vi "_builtins_arrange_object.vi"(8 "error in (no error)":errorcluster, 10 "Arrange":T1, 11 "GObject in":refnum<vi>) -> (0 "error out":errorcluster, 2 "object arranged?":bool, 3 "GObject out":refnum<vi>)   [LabVIEW 2019, in "Script.lvlib"]
doc: "Arranges the selected block diagram objects vertically to align the source terminal to the adjacent sink terminal (left-to-right) or sink to source terminals (right-to-left).\n\nCreated by: Ryan Pacini"
uses:
  Script.lvlib
  _builtins_arrange.ctl
  _builtins_label_position.ctl
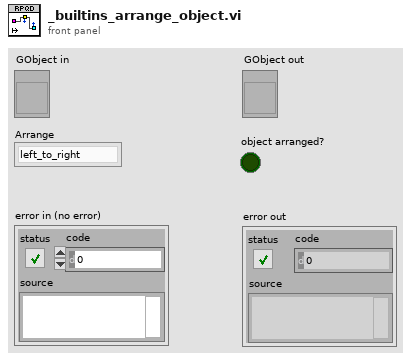
[diagram p1: front panel]
types:
  T1 = typedef "Script.lvlib/_builtins_arrange.ctl" = enum8{"left_to_right", "right_to_left"}
  T2 = typedef "Script.lvlib/_builtins_label_position.ctl" = enum8{"Unchanged", "Top-left", "Top-middle", "Top-right", "Right-top", "Right-middle", "Right-bottom", "Bottom-right", "Bottom-middle", "Bottom-left", "Left-bottom", "Left-middle", "Left-top"}
  T3 = typedef "LVRectTypeDef.ctl" = cluster{"Left":i16, "Top":i16, "Right":i16, "Bottom":i16}
  T4 = cluster{"Position":cluster{"h":i16, "v":i16}, "Flags":i32, "Type":enum32{"LooseEnd", "Endpoint", "Bend", "Junction"}, "Up Joint Index":i16, "Down Joint Index":i16, "Left Joint Index":i16, "Right Joint Index":i16}[]
  T5 = typedef "LVPositionTypeDef.ctl" = cluster{"Left":i32, "Top":i32}
  T6 = cluster{"Left":i32, "Top":i32, "Right":i32, "Bottom":i32}
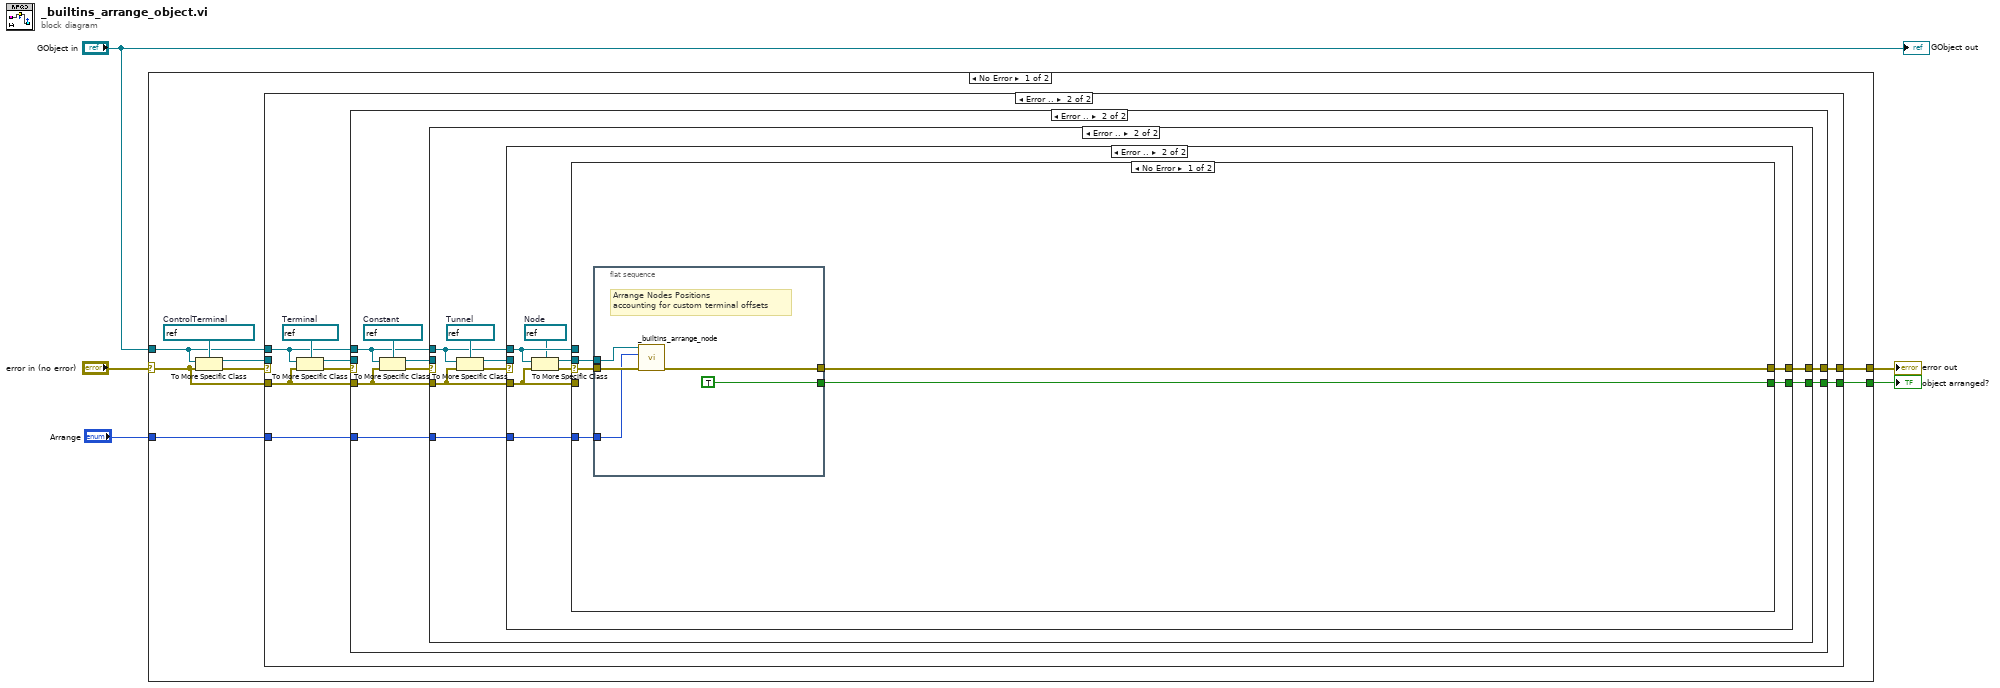
[diagram p0: block diagram]
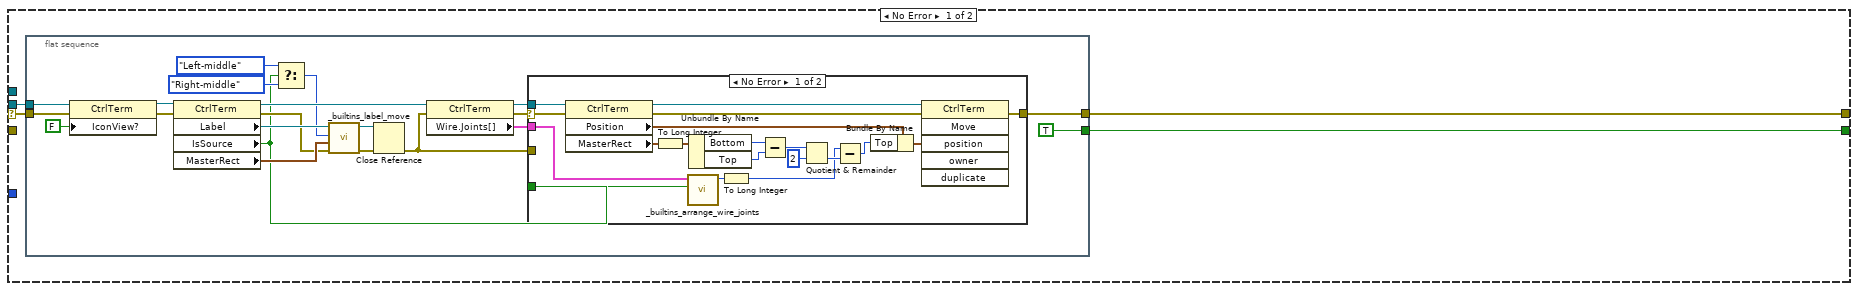
[diagram p2: hidden frame]
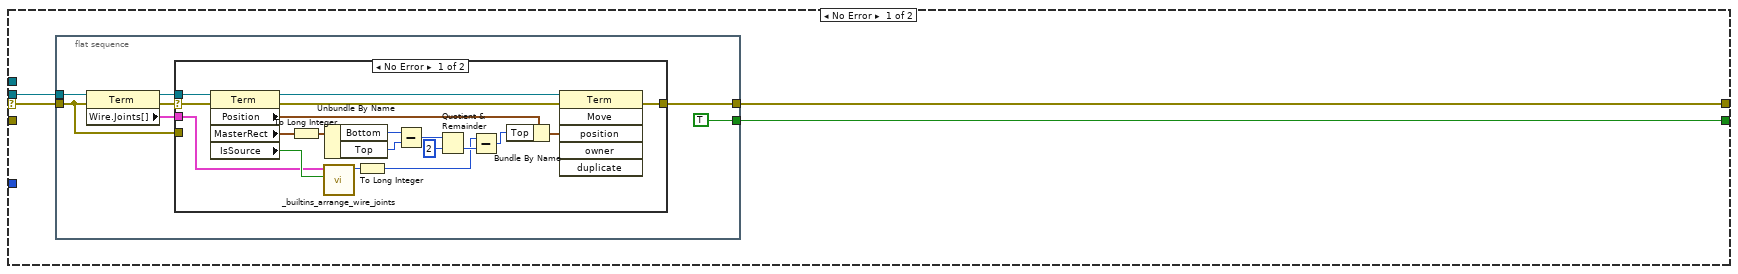
[diagram p4: hidden frame]
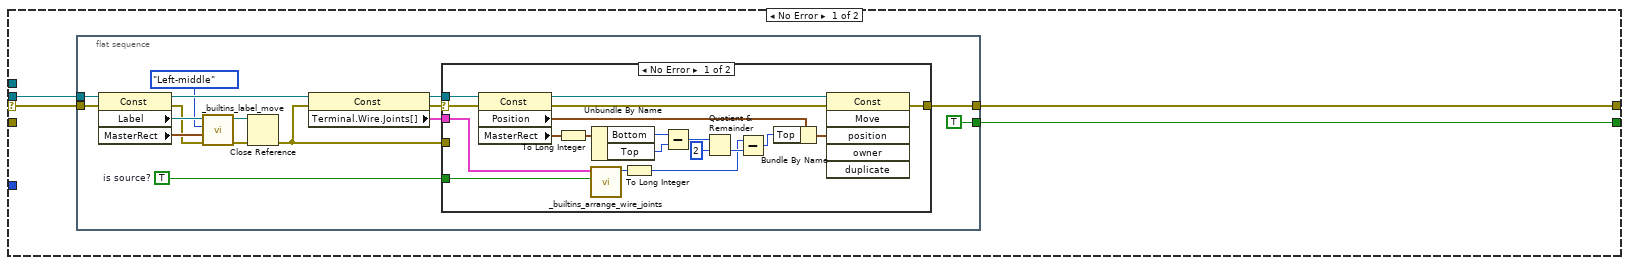
[diagram p6: hidden frame]
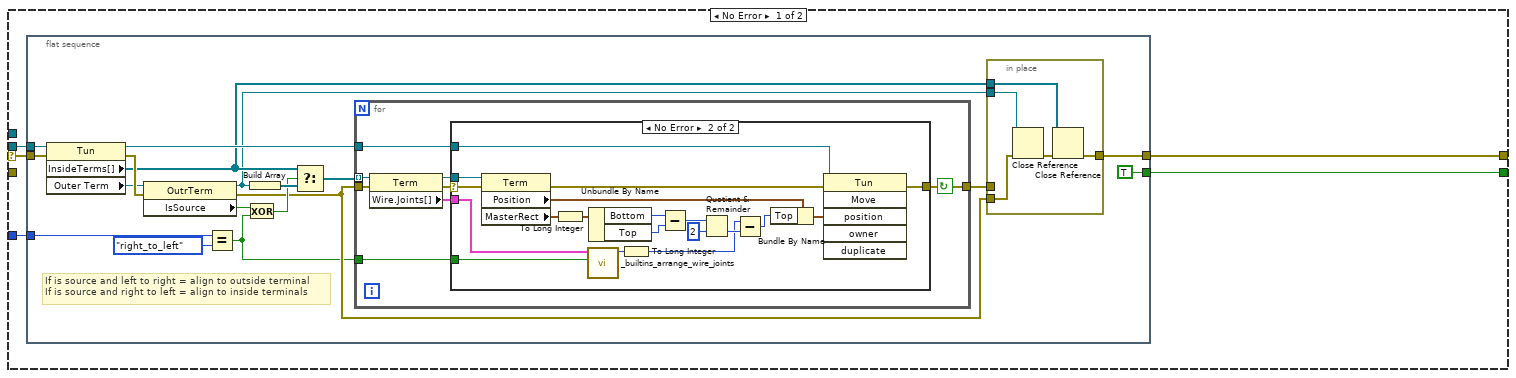
[diagram p8: hidden frame]
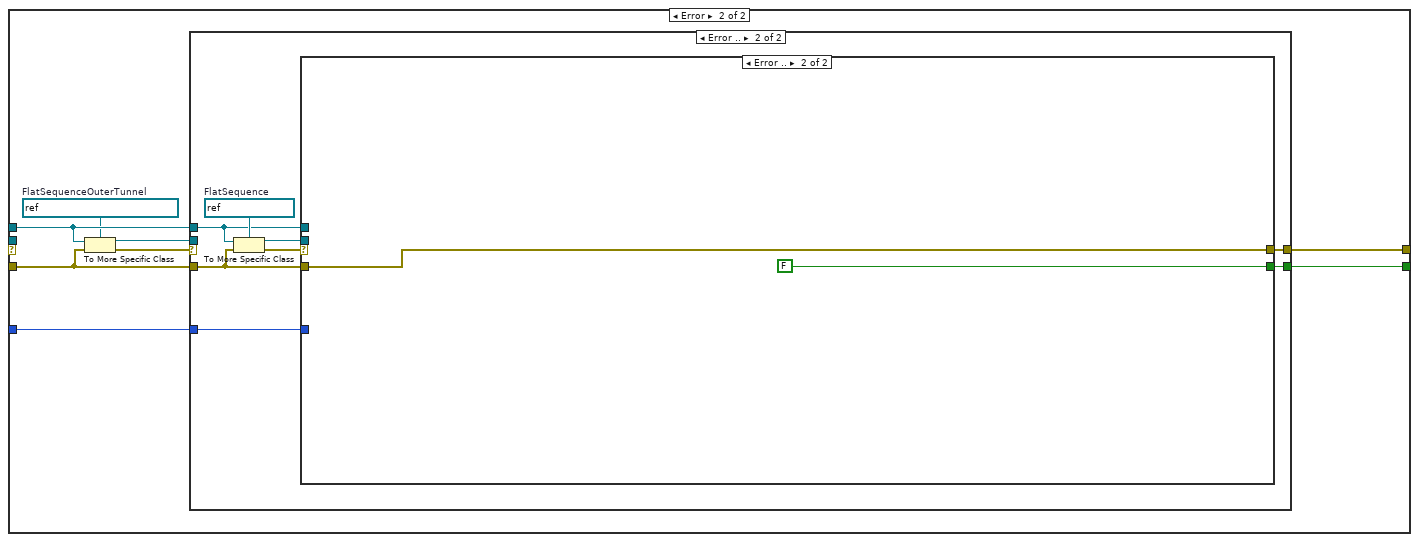
[diagram p10: hidden frame]
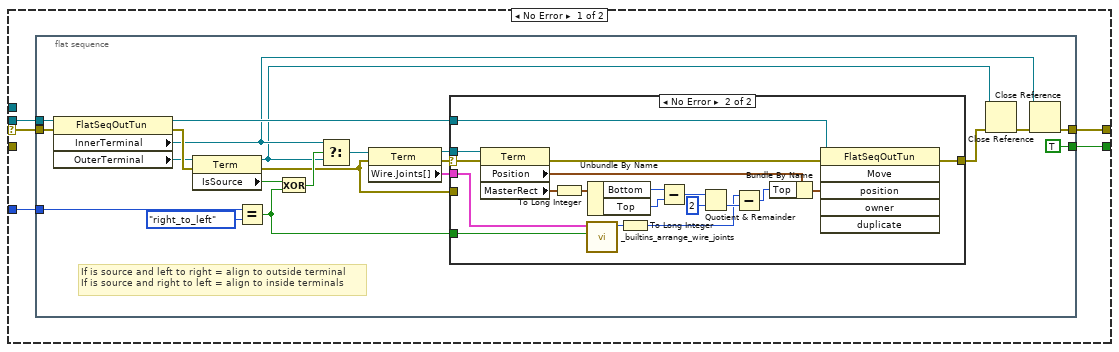
[diagram p11: hidden frame]
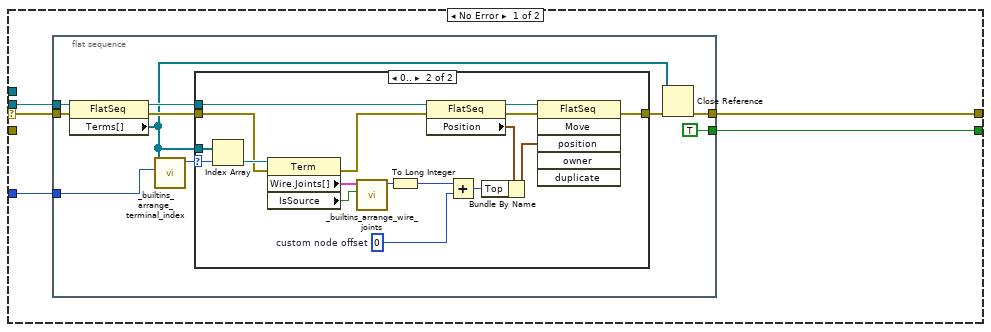
[diagram p13: hidden frame]
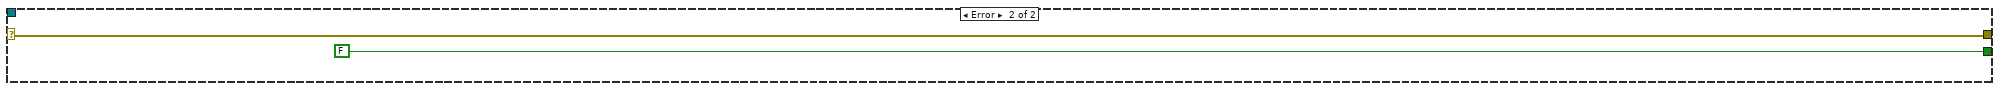
[diagram p15: hidden frame]
diagram:
  n1 = case shown="No Error" "error in (no error)" {
    selector: "error in (no error)" -> [w10 w326]
    tunnel: "GObject in" -> [w9 _]
    tunnel: [w8 w326] -> w3
    tunnel: [w7 FALSE] -> w1
    tunnel: "Arrange" -> [w6 _]
    frame No Error {
      w13 = refnum<vi> refnum  # ControlTerminal
      n2 = To More Specific Class(target class=w13, reference=w9, error in=w10) -> (specific class reference=w11:refnum<vi>, error out=w12:errorcluster)
      n3 = case shown="Error .." w12 {
        selector: w12 -> [w17 _]
        tunnel: w11 -> [w16 _]
        tunnel: [w15 w61] -> w8
        tunnel: w10 -> [_ w63]
        tunnel: w9 -> [_ w62]
        tunnel: w6 -> [_ w60]
        tunnel: [w14 w59] -> w7
        frame No Error {
          n4 = flat-sequence {
            tunnel: w17 -> [w38]
            tunnel: w16 -> [w37]
            tunnel: [w27] -> w15
            tunnel: [TRUE] -> w14
            frame #0 {
              n5 = property class="CtrlTerm"(reference=w37, error in=w38, "IconView?"=FALSE ("Icon View?")) -> (reference out=w34:refnum<vi>, error out=w35:errorcluster)
              n6 = property class="CtrlTerm"(reference=w34, error in=w35) -> (reference out=w28:refnum<vi>, error out=w31:errorcluster, "Label"=w33:refnum<vi>, "IsSource"=w19:bool, "MasterRect"=w32:T3)
              n7 = Select(t=_builtins_label_position."Left-middle" ("Label Position"), s=w19, f=_builtins_label_position."Right-middle" ("Label Position")) -> (s? t:f=w18:T2)
              n8 = call "_builtins_label_move.vi"("error in (no error)"=w31, "Owner Master Bounds Rect"=w32, "Label Position"=w18, "Label in"=w33) -> ("error out"=w30:errorcluster, "dup Label"=w29:refnum<vi>)  [unwired: 6 in]
              n9 = Close Reference(reference=w29, error in (no error)=w30) -> (error out=w22:errorcluster)
              n10 = property class="CtrlTerm"(reference=w28, error in=w22) -> (reference out=w25:refnum<vi>, error out=w24:errorcluster, "Wire.Joints[]"=w23:T4)
              n11 = case shown="No Error" w24 {
                selector: w24 -> [w40 _]
                tunnel: w19 -> [w45 _]
                tunnel: [w42 w58] -> w27
                tunnel: w25 -> [w41 _]
                tunnel: w23 -> [w39 _]
                tunnel: w22 -> [_ w58]
                frame No Error {
                  n12 = property class="CtrlTerm"(reference=w41, error in=w40) -> (reference out=w57:refnum<vi>, error out=w56:errorcluster, "Position"=w55:T5, "MasterRect"=w53:T3)
                  n13 = To Long Integer(number=w53) -> (32bit integer=w50:T6)
                  n14 = call "_builtins_arrange_wire_joints.vi"("Is Source?"=w45, "Joints"=w39) -> ("Vertical Position"=w44:i16)  [unwired: 8 in, 1 out]
                  n15 = Unbundle By Name(w50) -> ("Bottom"=w52:i32, "Top"=w51:i32)
                  n16 = To Long Integer(number=w44) -> (32bit integer=w43:i32)
                  n17 = Subtract(x=w52, y=w51) -> (x-y=w49:i32)
                  n18 = Quotient & Remainder(x=w49, y=2) -> (floor(x/y)=w47:i32)  [unwired: 1 out]
                  n19 = Subtract(x=w43, y=w47) -> (x-y=w46:i32)
                  n20 = Bundle By Name(cluster=w55, "Top"=w46) -> (w54:T5)
                  n21 = invoke class="CtrlTerm" method="Move"(reference=w57, error in=w56, "position"=w54) -> (error out=w42:errorcluster)  [unwired: 3 in, 5 out]
                }
                frame Error {
                }
              }
            }
          }
        }
        frame Error {
          w66 = refnum<vi> refnum  # Terminal
          n22 = To More Specific Class(target class=w66, reference=w62, error in=w63) -> (specific class reference=w64:refnum<vi>, error out=w65:errorcluster)
          n23 = case shown="Error .." w65 {
            selector: w65 -> [w70 _]
            tunnel: w64 -> [w69 _]
            tunnel: w63 -> [_ w101]
            tunnel: w62 -> [_ w102]
            tunnel: [w68 w100] -> w61
            tunnel: w60 -> [_ w99]
            tunnel: [w67 w98] -> w59
            frame No Error {
              n24 = flat-sequence {
                tunnel: w70 -> [w71]
                tunnel: w69 -> [w76]
                tunnel: [w77] -> w68
                tunnel: [TRUE] -> w67
                frame #0 {
                  n25 = property class="Term"(reference=w76, error in=w71) -> (reference out=w74:refnum<vi>, error out=w73:errorcluster, "Wire.Joints[]"=w72:T4)
                  n26 = case shown="No Error" w73 {
                    selector: w73 -> [w79 _]
                    tunnel: [w82 w97] -> w77
                    tunnel: w74 -> [w80 _]
                    tunnel: w72 -> [w78 _]
                    tunnel: w71 -> [_ w97]
                    frame No Error {
                      n27 = property class="Term"(reference=w80, error in=w79) -> (reference out=w96:refnum<vi>, error out=w95:errorcluster, "Position"=w94:T5, "MasterRect"=w92:T3, "IsSource"=w81:bool)
                      n28 = To Long Integer(number=w92) -> (32bit integer=w89:T6)
                      n29 = call "_builtins_arrange_wire_joints.vi"("Is Source?"=w81, "Joints"=w78) -> ("Vertical Position"=w84:i16)  [unwired: 8 in, 1 out]
                      n30 = Unbundle By Name(w89) -> ("Bottom"=w91:i32, "Top"=w90:i32)
                      n31 = To Long Integer(number=w84) -> (32bit integer=w83:i32)
                      n32 = Subtract(x=w91, y=w90) -> (x-y=w88:i32)
                      n33 = Quotient & Remainder(x=w88, y=2) -> (floor(x/y)=w86:i32)  [unwired: 1 out]
                      n34 = Subtract(x=w83, y=w86) -> (x-y=w85:i32)
                      n35 = Bundle By Name(cluster=w94, "Top"=w85) -> (w93:T5)
                      n36 = invoke class="Term" method="Move"(reference=w96, error in=w95, "position"=w93) -> (error out=w82:errorcluster)  [unwired: 3 in, 5 out]
                    }
                    frame Error {
                    }
                  }
                }
              }
            }
            frame Error {
              w105 = refnum<vi> refnum  # Constant
              n37 = To More Specific Class(target class=w105, reference=w102, error in=w101) -> (specific class reference=w103:refnum<vi>, error out=w104:errorcluster)
              n38 = case shown="Error .." w104 {
                selector: w104 -> [w109 _]
                tunnel: w103 -> [w108 _]
                tunnel: w102 -> [_ w149]
                tunnel: w101 -> [_ w150]
                tunnel: [w107 w147] -> w100
                tunnel: w99 -> [_ w148]
                tunnel: [w106 w146] -> w98
                frame No Error {
                  n39 = flat-sequence {
                    tunnel: w109 -> [w117]
                    tunnel: w108 -> [w118]
                    tunnel: [w120] -> w107
                    tunnel: [TRUE] -> w106
                    frame #0 {
                      w119 = TRUE  # is source?
                      n40 = property class="Const"(reference=w118, error in=w117) -> (reference out=w114:refnum<vi>, error out=w123:errorcluster, "Label"=w125:refnum<vi>, "MasterRect"=w124:T3)
                      n41 = call "_builtins_label_move.vi"("error in (no error)"=w123, "Owner Master Bounds Rect"=w124, "Label Position"=_builtins_label_position."Left-middle", "Label in"=w125) -> ("error out"=w122:errorcluster, "dup Label"=w121:refnum<vi>)  [unwired: 6 in]
                      n42 = Close Reference(reference=w121, error in (no error)=w122) -> (error out=w111:errorcluster)
                      n43 = property class="Const"(reference=w114, error in=w111) -> (reference out=w115:refnum<vi>, error out=w112:errorcluster, "Terminal.Wire.Joints[]"=w113:T4)
                      n44 = case shown="No Error" w112 {
                        selector: w112 -> [w126 _]
                        tunnel: [w130 w145] -> w120
                        tunnel: w119 -> [w129 _]
                        tunnel: w115 -> [w128 _]
                        tunnel: w113 -> [w127 _]
                        tunnel: w111 -> [_ w145]
                        frame No Error {
                          n45 = property class="Const"(reference=w128, error in=w126) -> (reference out=w144:refnum<vi>, error out=w143:errorcluster, "Position"=w142:T5, "MasterRect"=w140:T3)
                          n46 = To Long Integer(number=w140) -> (32bit integer=w137:T6)
                          n47 = call "_builtins_arrange_wire_joints.vi"("Is Source?"=w129, "Joints"=w127) -> ("Vertical Position"=w132:i16)  [unwired: 8 in, 1 out]
                          n48 = Unbundle By Name(w137) -> ("Bottom"=w139:i32, "Top"=w138:i32)
                          n49 = To Long Integer(number=w132) -> (32bit integer=w131:i32)
                          n50 = Subtract(x=w139, y=w138) -> (x-y=w136:i32)
                          n51 = Quotient & Remainder(x=w136, y=2) -> (floor(x/y)=w134:i32)  [unwired: 1 out]
                          n52 = Subtract(x=w131, y=w134) -> (x-y=w133:i32)
                          n53 = Bundle By Name(cluster=w142, "Top"=w133) -> (w141:T5)
                          n54 = invoke class="Const" method="Move"(reference=w144, error in=w143, "position"=w141) -> (error out=w130:errorcluster)  [unwired: 3 in, 5 out]
                        }
                        frame Error {
                        }
                      }
                    }
                  }
                }
                frame Error {
                  w153 = refnum<vi> refnum  # Tunnel
                  n55 = To More Specific Class(target class=w153, reference=w149, error in=w150) -> (specific class reference=w151:refnum<vi>, error out=w152:errorcluster)
                  n56 = case shown="Error .." w152 {
                    selector: w152 -> [w158 _]
                    tunnel: w151 -> [w157 _]
                    tunnel: w150 -> [_ w214]
                    tunnel: w149 -> [_ w215]
                    tunnel: w148 -> [w156 w213]
                    tunnel: [w155 w212] -> w147
                    tunnel: [w154 w211] -> w146
                    frame No Error {
                      n57 = flat-sequence {
                        tunnel: w158 -> [w176]
                        tunnel: w157 -> [w175]
                        tunnel: w156 -> [w161]
                        tunnel: [w165] -> w155
                        tunnel: [TRUE] -> w154
                        frame #0 {
                          # "If is source and left to right = align to outside terminal\nIf is source and right to left = align to inside terminals"
                          n58 = property class="Tun"(reference=w175, error in=w176) -> (reference out=w168:refnum<vi>, error out=w174:errorcluster, "InsideTerms[]"=w167:refnum<vi>[], "Outer Term"=w173:refnum<vi>)
                          n59 = property class="OutrTerm"(reference=w173, error in=w174) -> (reference out=w166:refnum<vi>, error out=w163:errorcluster, "IsSource"=w171:bool)
                          n60 = Equal?(x=w161, y=_builtins_arrange."right_to_left" ("Arrange")) -> (x = y?=w159:bool)
                          n61 = Exclusive Or(1:w159, 2:w171) -> (0:w170:bool)
                          n62 = Build Array(w166) -> (w172:refnum<vi>[])
                          n63 = Select(t=w167, s=w170, f=w172) -> (s? t:f=w169:refnum<vi>[])
                          n64 = for {
                            tunnel: w169 -> [w189] mode=indexing
                            tunnel: w159 -> [w187]
                            tunnel: w163 -> [w186]
                            tunnel: w168 -> [w185]
                            tunnel: [w182] -> w164
                            stop <- w182 continue-if-true
                            n65 = property class="Term"(reference=w189, error in=w186) -> (reference out=w183:refnum<vi>, error out=w188:errorcluster, "Wire.Joints[]"=w184:T4)
                            n66 = case shown="No Error" w188 {
                              selector: w188 -> [w190 w196]
                              tunnel: w187 -> [_ w197]
                              tunnel: [w190 w194] -> w182
                              tunnel: w185 -> [_ w193]
                              tunnel: w184 -> [_ w191]
                              tunnel: w183 -> [_ w192]
                              frame Error {
                              }
                              frame No Error {
                                n67 = property class="Term"(reference=w192, error in=w196) -> (error out=w195:errorcluster, "Position"=w199:T5, "MasterRect"=w200:T3)  [unwired: 1 out]
                                n68 = To Long Integer(number=w200) -> (32bit integer=w207:T6)
                                n69 = call "_builtins_arrange_wire_joints.vi"("Is Source?"=w197, "Joints"=w191) -> ("Vertical Position"=w202:i16)  [unwired: 8 in, 1 out]
                                n70 = Unbundle By Name(w207) -> ("Bottom"=w209:i32, "Top"=w208:i32)
                                n71 = To Long Integer(number=w202) -> (32bit integer=w201:i32)
                                n72 = Subtract(x=w209, y=w208) -> (x-y=w206:i32)
                                n73 = Quotient & Remainder(x=w206, y=2) -> (floor(x/y)=w204:i32)  [unwired: 1 out]
                                n74 = Subtract(x=w201, y=w204) -> (x-y=w203:i32)
                                n75 = Bundle By Name(cluster=w199, "Top"=w203) -> (w198:T5)
                                n76 = invoke class="Tun" method="Move"(reference=w193, error in=w195, "position"=w198) -> (error out=w194:errorcluster)  [unwired: 3 in, 5 out]
                              }
                            }
                          }
                          n77 = in-place {
                            in-place-border: w167 -> [w181]
                            in-place-border: w164 -> [_]
                            in-place-border: w166 -> [w179]
                            in-place-border: [w178] -> w165
                            in-place-border: w163 -> [w177]
                            n78 = Close Reference(reference=w179, error in (no error)=w177) -> (error out=w180:errorcluster)
                            n79 = Close Reference(reference=w181, error in (no error)=w180) -> (error out=w178:errorcluster)
                          }
                        }
                      }
                    }
                    frame Error {
                      w210 = refnum<vi> refnum  # Node
                      n80 = To More Specific Class(target class=w210, reference=w215, error in=w214) -> (specific class reference=w216:refnum<vi>, error out=w217:errorcluster)
                      n81 = case shown="No Error" w217 {
                        selector: w217 -> [w222 _]
                        tunnel: w216 -> [w221 _]
                        tunnel: w215 -> [_ w233]
                        tunnel: w214 -> [_ w232]
                        tunnel: w213 -> [w220 w229]
                        tunnel: [w219 w231] -> w212
                        tunnel: [w218 w230] -> w211
                        frame No Error {
                          n82 = flat-sequence {
                            tunnel: [TRUE] -> w218
                            tunnel: w221 -> [w225]
                            tunnel: w222 -> [w226]
                            tunnel: w220 -> [w224]
                            tunnel: [w223] -> w219
                            frame #0 {
                              # "Arrange Nodes Positions\naccounting for custom terminal offsets"
                              n83 = call "_builtins_arrange_node.vi"("error in (no error)"=w226, "Arrange"=w224, "Node in"=w225) -> ("error out"=w223:errorcluster)  [unwired: 7 in, 1 out]
                            }
                          }
                        }
                        frame Error {
                          w228 = refnum<vi> refnum  # FlatSequenceOuterTunnel
                          n84 = To More Specific Class(target class=w228, reference=w233, error in=w232) -> (specific class reference=w234:refnum<vi>, error out=w235:errorcluster)
                          n85 = case shown="Error .." w235 {
                            selector: w235 -> [w238 _]
                            tunnel: w234 -> [w237 _]
                            tunnel: w233 -> [_ w286]
                            tunnel: w232 -> [_ w287]
                            tunnel: [w239 w284] -> w231
                            tunnel: [w240 w283] -> w230
                            tunnel: w229 -> [w236 w282]
                            frame No Error {
                              n86 = flat-sequence {
                                tunnel: w238 -> [w261]
                                tunnel: w237 -> [w260]
                                tunnel: w236 -> [w254]
                                tunnel: [w249] -> w239
                                tunnel: [TRUE] -> w240
                                frame #0 {
                                # "If is source and left to right = align to outside terminal\nIf is source and right to left = align to inside terminals"
                                n87 = property class="FlatSeqOutTun"(reference=w260, error in=w261) -> (reference out=w253:refnum<vi>, error out=w259:errorcluster, "InnerTerminal"=w252:refnum<vi>, "OuterTerminal"=w258:refnum<vi>)
                                n88 = property class="Term"(reference=w258, error in=w259) -> (reference out=w245:refnum<vi>, error out=w244:errorcluster, "IsSource"=w257:bool)
                                n89 = Equal?(x=w254, y=_builtins_arrange."right_to_left" ("Arrange")) -> (x = y?=w241:bool)
                                n90 = Exclusive Or(1:w241, 2:w257) -> (0:w256:bool)
                                n91 = Select(t=w252, s=w256, f=w245) -> (s? t:f=w255:refnum<vi>)
                                n92 = property class="Term"(reference=w255, error in=w244) -> (reference out=w246:refnum<vi>, error out=w248:errorcluster, "Wire.Joints[]"=w247:T4)
                                n93 = case shown="No Error" w248 {
                                selector: w248 -> [_ w268]
                                tunnel: w241 -> [_ w269]
                                tunnel: [w262 w266] -> w251
                                tunnel: w253 -> [_ w265]
                                tunnel: w247 -> [_ w263]
                                tunnel: w246 -> [_ w264]
                                tunnel: w244 -> [w262 _]
                                frame Error {
                                }
                                frame No Error {
                                n94 = property class="Term"(reference=w264, error in=w268) -> (error out=w267:errorcluster, "Position"=w271:T5, "MasterRect"=w272:T3)  [unwired: 1 out]
                                n95 = To Long Integer(number=w272) -> (32bit integer=w279:T6)
                                n96 = call "_builtins_arrange_wire_joints.vi"("Is Source?"=w269, "Joints"=w263) -> ("Vertical Position"=w274:i16)  [unwired: 8 in, 1 out]
                                n97 = Unbundle By Name(w279) -> ("Bottom"=w281:i32, "Top"=w280:i32)
                                n98 = To Long Integer(number=w274) -> (32bit integer=w273:i32)
                                n99 = Subtract(x=w281, y=w280) -> (x-y=w278:i32)
                                n100 = Quotient & Remainder(x=w278, y=2) -> (floor(x/y)=w276:i32)  [unwired: 1 out]
                                n101 = Subtract(x=w273, y=w276) -> (x-y=w275:i32)
                                n102 = Bundle By Name(cluster=w271, "Top"=w275) -> (w270:T5)
                                n103 = invoke class="FlatSeqOutTun" method="Move"(reference=w265, error in=w267, "position"=w270) -> (error out=w266:errorcluster)  [unwired: 3 in, 5 out]
                                }
                                }
                                n104 = Close Reference(reference=w245, error in (no error)=w251) -> (error out=w250:errorcluster)
                                n105 = Close Reference(reference=w252, error in (no error)=w250) -> (error out=w249:errorcluster)
                                }
                              }
                            }
                            frame Error {
                              w289 = refnum<vi> refnum  # FlatSequence
                              n106 = To More Specific Class(target class=w289, reference=w286, error in=w287) -> (specific class reference=w285:refnum<vi>, error out=w288:errorcluster)
                              n107 = case shown="Error .." w288 {
                                selector: w288 -> [w294 _]
                                tunnel: w287 -> [_ w324]
                                tunnel: w286 -> [_ _]
                                tunnel: w285 -> [w293 _]
                                tunnel: [w290 w324] -> w284
                                tunnel: [w291 FALSE] -> w283
                                tunnel: w282 -> [w292 _]
                                frame No Error {
                                n108 = flat-sequence {
                                tunnel: [TRUE] -> w291
                                tunnel: w293 -> [w303]
                                tunnel: w294 -> [w301]
                                tunnel: w292 -> [w298]
                                tunnel: [w296] -> w290
                                frame #0 {
                                n109 = property class="FlatSeq"(reference=w303, error in=w301) -> (reference out=w302:refnum<vi>, error out=w300:errorcluster, "Terms[]"=w295:refnum<vi>[])
                                n110 = call "_builtins_arrange_terminal_index.vi"("Arrange"=w298, "Terminals"=w295) -> ("Terminal Index"=w299:i32)  [unwired: 9 in]
                                n111 = case shown="0.." w299 {
                                selector: w299 -> [_ w310]
                                tunnel: [w305 w322] -> w297
                                tunnel: w302 -> [_ w317]
                                tunnel: w300 -> [w305 w306]
                                tunnel: w295 -> [_ w311]
                                frame ..-1 {
                                }
                                frame 0.. {
                                w309 = 0  # custom node offset
                                n112 = Index Array(array=w311, index=w310) -> (element=w308:refnum<vi>)
                                n113 = property class="Term"(reference=w308, error in=w306) -> (error out=w307:errorcluster, "Wire.Joints[]"=w313:T4, "IsSource"=w312:bool)  [unwired: 1 out]
                                n114 = call "_builtins_arrange_wire_joints.vi"("Is Source?"=w312, "Joints"=w313) -> ("Vertical Position"=w316:i16)  [unwired: 8 in, 1 out]
                                n115 = To Long Integer(number=w316) -> (32bit integer=w314:i32)
                                n116 = property class="FlatSeq"(reference=w317, error in=w307) -> (reference out=w320:refnum<vi>, error out=w321:errorcluster, "Position"=w319:T5)
                                n117 = Add(x=w314, y=w309) -> (x+y=w315:i32)
                                n118 = Bundle By Name(cluster=w319, "Top"=w315) -> (w318:T5)
                                n119 = invoke class="FlatSeq" method="Move"(reference=w320, error in=w321, "position"=w318) -> (error out=w322:errorcluster)  [unwired: 3 in, 5 out]
                                }
                                }
                                n120 = Close Reference(reference=w295, error in (no error)=w297) -> (error out=w296:errorcluster)
                                }
                                }
                                }
                                frame Error {
                                }
                              }
                            }
                          }
                        }
                      }
                    }
                  }
                }
              }
            }
          }
        }
      }
    }
    frame Error {
    }
  }
  "error out" <- w3
  "object arranged?" <- w1
  "GObject out" <- "GObject in"
